vi "Default Test Result.vi"() -> (3 "TestStand Result":T1)   [LabVIEW 2020, in "Report CSV Content Test.lvclass"]
uses:
  Report CSV Content Test.lvclass
  source/Test Result Handler/TestStand Result.ctl
  source/Test Result Handler/TestStand Result Handler.lvclass
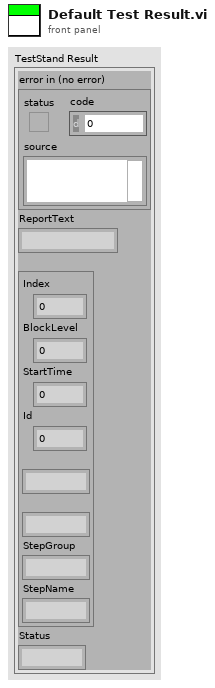
[diagram p1: front panel]
types:
  T1 = typedef "Astemes_CSVReportPlugin.lvlib/TestStand Result Handler.lvclass/TestStand Result.ctl" = cluster{"error in (no error)":errorcluster, "ReportText":string, "TS":cluster{"Index":i32, "BlockLevel":i32, "StartTime":dbl, "Id":i32, "StepType":string, "StepID":string, "StepGroup":string, "StepName":string}, "Status":string}
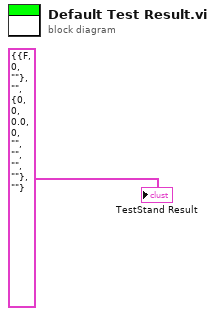
[diagram p0: block diagram]
diagram:
  "TestStand Result" <- T1 {"error in (no error)"={"status"=FALSE, "code"=0, "source"=""}, "ReportText"="", "TS"={"Index"=0, "BlockLevel"=0, "StartTime"=0.0, "Id"=0, "StepType"="", "StepID"="", "StepGroup"="", "StepName"=""}, "Status"=""} ("TestStand Result")
